vi "Accessory.vi"() -> ()   [LabVIEW 2011]
panel:
  in  "Sound?":bool
  out "Time":dbl
  in  "Start Timer":bool
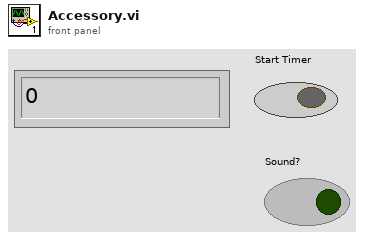
[diagram p1: front panel]
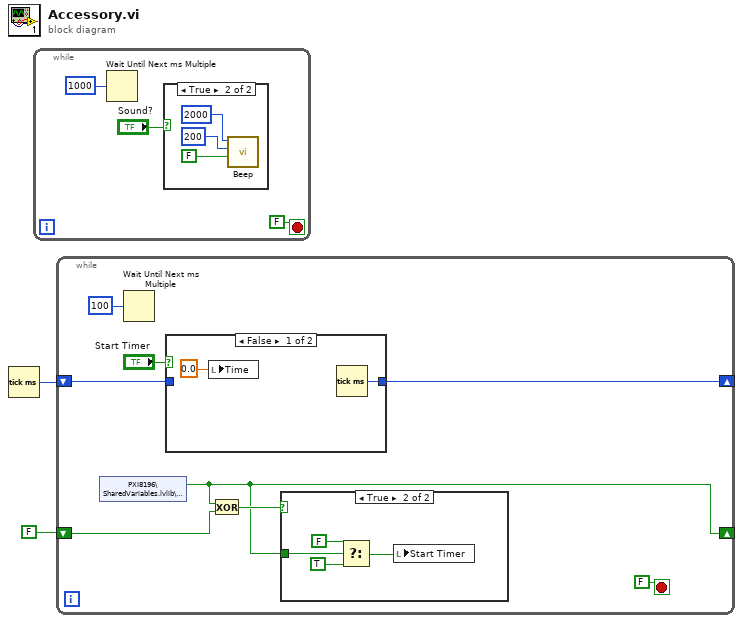
[diagram p0: block diagram]
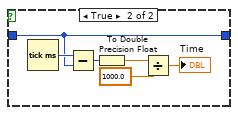
[diagram p3: hidden frame]
diagram:
  n1 = Tick Count (ms)() -> (millisecond timer value=w2:u32)
  n2 = while {
    stop <- FALSE stop-if-true
    n3 = Wait Until Next ms Multiple(millisecond multiple=u32 1000) -> ()  [unwired: 1 out]
    n4 = case shown="True" "Sound?" {
      frame False {
      }
      frame True {
        n5 = call <vilib>:"Beep.vi"("use system alert? (T)"=FALSE, "duration (msec)"=u32 200, "frequency (Hz)"=u32 2000) -> ()  [unwired: 9 in]
      }
    }
  }
  n6 = while {
    shift-right: [w14] -> _
    shift-left: w2 -> [w12]
    shift-right: [w9] -> _
    shift-left: FALSE -> [w11]
    stop <- FALSE stop-if-true
    n7 = shared-variable "PXI8196\\SharedVariables.lvlib\\Record?"() -> (w9:bool)  [unwired: 1 in, 1 out]
    n8 = Wait Until Next ms Multiple(millisecond multiple=u32 100) -> ()  [unwired: 1 out]
    n9 = case shown="False" "Start Timer" {
      tunnel: [w22 w27] -> w14
      tunnel: w12 -> [_ w27]
      frame False {
        n10 = local write "Time"(0.0 ("Time")) -> ()
        n11 = Tick Count (ms)() -> (millisecond timer value=w22:u32)
      }
      frame True {
        n12 = Tick Count (ms)() -> (millisecond timer value=w28:u32)
        n13 = Subtract(x=w28, y=w27) -> (x-y=w24:u32)
        n14 = To Double Precision Float(number=w24) -> (double precision float=w25:dbl)
        n15 = Divide(x=w25, y=1000.0) -> (x/y=→"Time":dbl)
      }
    }
    n16 = Exclusive Or(1:w11, 2:w9) -> (0:w10:bool)
    n17 = case shown="True" w10 {
      tunnel: w9 -> [_ w20]
      frame False {
      }
      frame True {
        n18 = Select(t=FALSE, s=w20, f=TRUE) -> (s? t:f=w19:bool)
        n19 = local write "Start Timer"(w19) -> ()
      }
    }
  }
